vi "SLSC Change Color of Table Header.vi"(8 "error in (no error)":errorcluster, 10 "Active Cell:Active Column Number":i32=-3, 11 "TreeControl in":refnum<vi>) -> (0 "error out":errorcluster)   [LabVIEW 2015, in "SLSC Tree Control.lvlib"]
uses:
  SLSC Tree Control.lvlib
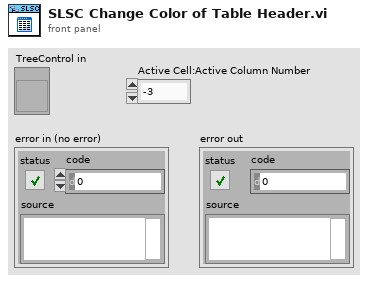
[diagram p1: front panel]
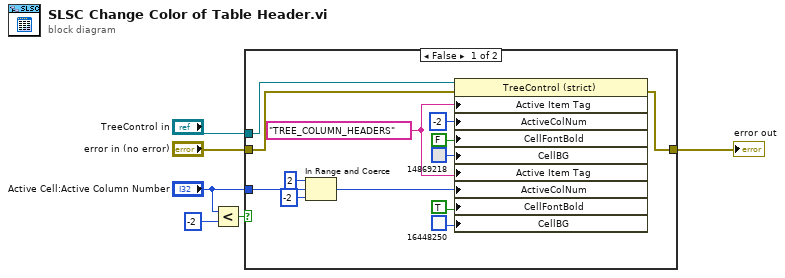
[diagram p0: block diagram]
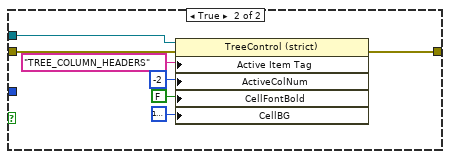
[diagram p2: hidden frame]
diagram:
  n1 = Less?(x="Active Cell:Active Column Number", y=-2) -> (x < y?=w4:bool)
  n2 = case shown="False" w4 {
    tunnel: "Active Cell:Active Column Number" -> [w13 _]
    tunnel: "error in (no error)" -> [w11 w23]
    tunnel: "TreeControl in" -> [w10 w22]
    tunnel: [w12 w21] -> w1
    frame False {
      w15 = "TREE_COLUMN_HEADERS" ("Active Item:Tag")
      n3 = In Range and Coerce(upper limit=2, x=w13, lower limit=-2) -> (coerced(x)=w9:i32)  [unwired: 1 out]
      n4 = property on="Property Node" class="TreeControl (strict)"(reference=w10, error in=w11, "Active Item Tag"=w15, "ActiveColNum"=-2 ("Active Cell:Active Column Number"), "CellFontBold"=FALSE ("Active Cell:Cell Font:Bold"), "CellBG"=u32 14869218 ("Color Box"), "Active Item Tag"=w15, "ActiveColNum"=w9, "CellFontBold"=TRUE ("Active Cell:Cell Font:Bold"), "CellBG"=u32 16448250 ("Color Box")) -> (error out=w12:errorcluster)  [unwired: 1 out]
    }
    frame True {
      n5 = property on="Property Node" class="TreeControl (strict)"(reference=w22, error in=w23, "Active Item Tag"="TREE_COLUMN_HEADERS" ("Active Item:Tag"), "ActiveColNum"=-2 ("Active Cell:Active Column Number"), "CellFontBold"=FALSE ("Active Cell:Cell Font:Bold"), "CellBG"=u32 16777238 ("Color Box")) -> (error out=w21:errorcluster)  [unwired: 1 out]
    }
  }
  "error out" <- w1
